vi "PDLM_SetLaserMode.vi"(8 "error in (no error)":errorcluster, 10 "mode":T1=enum."PULSE", 11 "USBIdx":i32) -> (0 "error out":errorcluster, 3 "return type":i32)   [LabVIEW 2019]
uses:
  <userlib>/TaikoLaser/PDLM_LaserMode.ctl
  <userlib>/TaikoLaser/PDLM_DllPath_global.vi
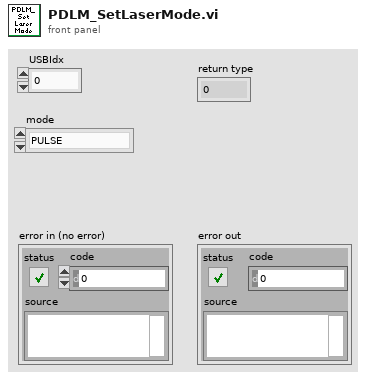
[diagram p1: front panel]
types:
  T1 = typedef "PDLM_LaserMode.ctl" = enum32{"CW", "PULSE", "BURST"}
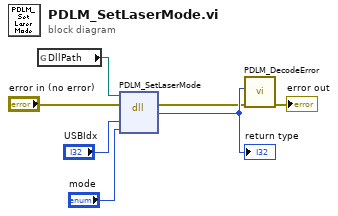
[diagram p0: block diagram]
diagram:
  n1 = global read "PDLM_DllPath_global.vi" "DllPath"() -> (w3:path)
  n2 = dll-call lib="M:/_dev/progs/LabVIEW/_lib/PQ/Taiko/pdlm_lib.dll" fn="PDLM_SetLaserMode"(path in=w3, error in="error in (no error)", "USBIdx"="USBIdx", "mode"="mode") -> (error out=w5:errorcluster, "return type"=w6:i32)  [unwired: 3 in, 1 out]
  "return type" <- w6
  n3 = call <userlib>:"PDLM_DecodeError.vi"("error in (no error)"=w5, "code"=w6) -> ("error out"=→"error out":errorcluster)  [unwired: 7 in, 2 out]
